vi "Create CMD for Read from PLC.vi"(9 "length":i16, 10 "Start Address":i32, 11 "action":T1(ring)) -> (3 "concatenated string 2":string)   [LabVIEW 2015]
panel:
  in  "Command":string="00FF000A"
  out "concatenated string 2":string
  out "concatenated string":string
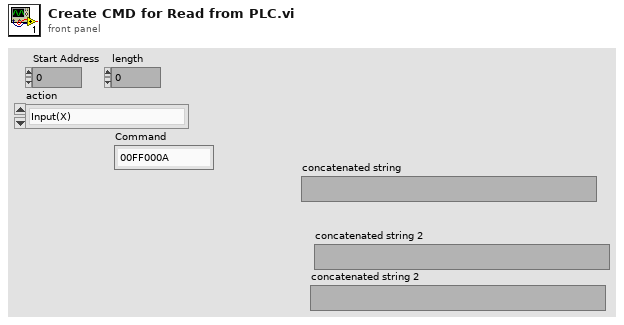
[diagram p1: front panel]
types:
  T1 = enum16{"Input(X)", "Output(Y)", "internal relay(M)", "Data Register(D)"}
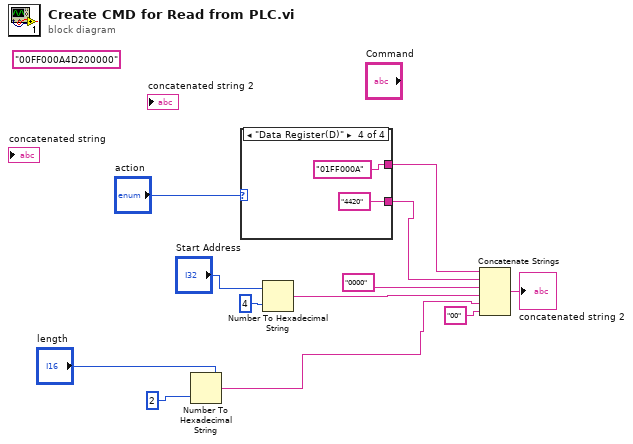
[diagram p0: block diagram]
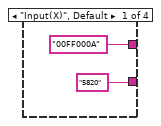
[diagram p2: hidden frame]
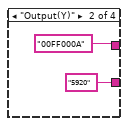
[diagram p3: hidden frame]
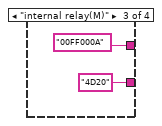
[diagram p4: hidden frame]
diagram:
  (unwired) "00FF000A4D200000" ("Command")
  n1 = Number To Hexadecimal String(1:i16 2 ("width (-)"), 2:"length") -> (0:w2:string)
  n2 = case shown="\"Data Register(D)\"" "action" {
    tunnel: ["5820" ("Command") "5920" ("Command") "4D20" ("Command") "4420" ("Command")] -> w7
    tunnel: ["00FF000A" ("Command") "00FF000A" ("Command") "00FF000A" ("Command") "01FF000A" ("Command")] -> w1
    frame "Input(X)", Default {
    }
    frame "Output(Y)" {
    }
    frame "internal relay(M)" {
    }
    frame "Data Register(D)" {
    }
  }
  n3 = Number To Hexadecimal String(1:i16 4 ("width (-)"), 2:"Start Address") -> (0:w10:string)
  n4 = Concatenate Strings(w1, w7, "0000" ("Command"), w10, w2, "00" ("Command")) -> (→"concatenated string 2":string)
